vi "Creador ruta archivo para lectura continua.vi"(4 "error in (no error)":errorcluster, 7 "Datos de Nueva Adquisición In":T1={"Equipo a Utilizar"=enum."TDS 2012B Osciloscope", "Montura"=enum."Motor Bipolar", "Datos Zaber"={"Sentido de Adquisición"=FALSE, "Comenzar Desde Home?"=FALSE, "Distancia a recorrer (um)"=0.0, "Pasos motor"=0, "Distancia entre Lecturas (um)"=0.0, "Puerto"=""}, "Datos Bipolar/Unipolar"={"Puerto COM"="", "Pasos entre Lecturas"=0, "Numero de lecturas"=0, "Sentido del motor"=TRUE}, "Datos Archivo"={"Ruta Archivo"=path "", "Nombre de Prueba"=""}, "Datos actuales"={"Montura"="", "Equipo"="", "Posición Actual"="", "Distancia Total a recorrer"="", "distancia Entre lecturas"="", "Pasos entre lecturas"=""}, "Datos a Guardar In"={"Datos Cursor Tektronix"="", "Datos Lokin"="", "Posición Cero"=0.0, "Posición Actual"=0.0}, "Datos Osciloscopio"={"Sesión Visa Osciloscopio"="Tektronix_TDS2012C", "Tipo de Adquisición"=enum."Voltaje Pico Pico", "Canal a Utilizar"=enum."Canal 1", "Parametros de Adquisición"=enum."Una Muestra", "Número Promedio"=2}, "Datos Lock In"={"Visa Lock in"="Tektronix_TDS2012C"}} {"Datos Osciloscopio"."Número Promedio" min=2 max=20; "Datos a Guardar In"."Posición Actual" format="%#_10f"; "Datos a Guardar In"."Posición Cero" format="%#_10f"; "Datos Bipolar/Unipolar"."Numero de lecturas" max=910098 step=1}) -> (0 "error out":errorcluster, 3 "Datos de Nueva Adquisición out":T1={"Equipo a Utilizar"=enum."TDS 2012B Osciloscope", "Montura"=enum."Motor Bipolar", "Datos Zaber"={"Sentido de Adquisición"=FALSE, "Comenzar Desde Home?"=FALSE, "Distancia a recorrer (um)"=0.0, "Pasos motor"=0, "Distancia entre Lecturas (um)"=0.0, "Puerto"=""}, "Datos Bipolar/Unipolar"={"Puerto COM"="", "Pasos entre Lecturas"=0, "Numero de lecturas"=0, "Sentido del motor"=TRUE}, "Datos Archivo"={"Ruta Archivo"=path "", "Nombre de Prueba"=""}, "Datos actuales"={"Montura"="", "Equipo"="", "Posición Actual"="", "Distancia Total a recorrer"="", "distancia Entre lecturas"="", "Pasos entre lecturas"=""}, "Datos a Guardar In"={"Datos Cursor Tektronix"="", "Datos Lokin"="", "Posición Cero"=0.0, "Posición Actual"=0.0}, "Datos Osciloscopio"={"Sesión Visa Osciloscopio"="Tektronix_TDS2012C", "Tipo de Adquisición"=enum."Voltaje Pico Pico", "Canal a Utilizar"=enum."Canal 1", "Parametros de Adquisición"=enum."Una Muestra", "Número Promedio"=2}, "Datos Lock In"={"Visa Lock in"="Tektronix_TDS2012C"}} {"Datos Osciloscopio"."Número Promedio" min=2 max=20; "Datos a Guardar In"."Posición Actual" format="%#_10f"; "Datos a Guardar In"."Posición Cero" format="%#_10f"; "Datos Bipolar/Unipolar"."Numero de lecturas" max=910098 step=1})   [LabVIEW 2020]
doc: "Este Vi Crea una ruta para el proyecto RPS utilizando fecha hora y nombre de prueba"
uses:
  Type Definitions/Asistente de adquisicion Cluster.ctl
  Type Definitions/Datos a Guardar.ctl
  Type Definitions/datos osciloscopio.ctl
  Type Definitions/Datos Zaber.ctl
  Type Definitions/parametros motores.ctl
  H:/Mi unidad/Departamento de Ingenieria/Investigadores/Gabriel Ramos/Proyecto Monturas v13/LV Source/Type Definitions/Tipos de montura.ctl
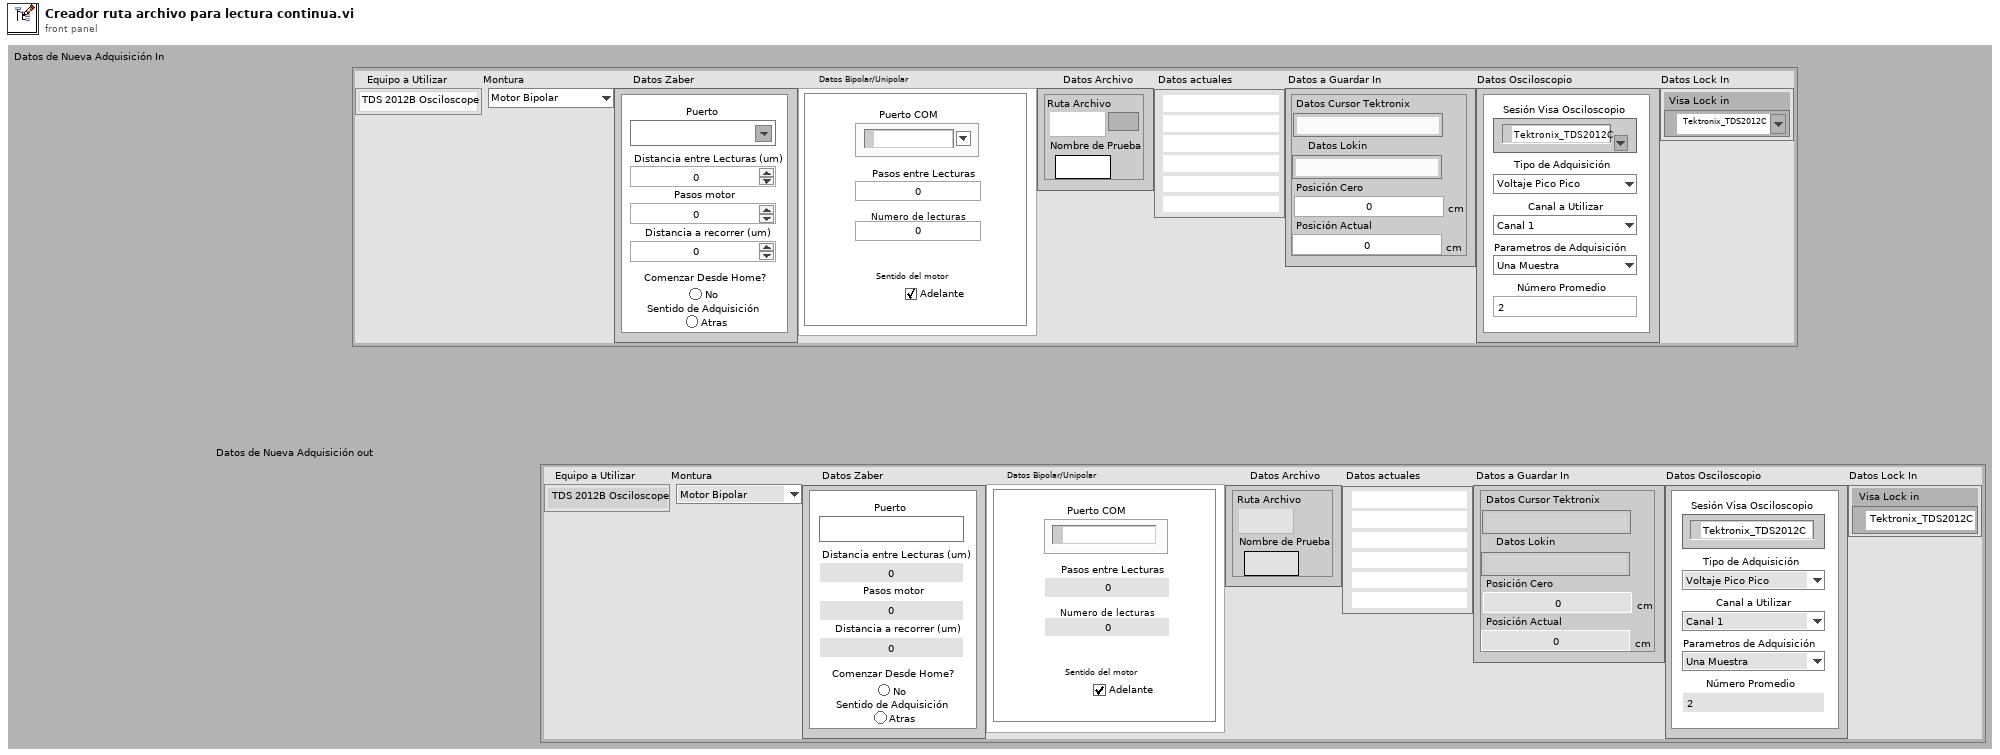
[diagram p1: front panel]
types:
  T1 = typedef "Asistente de adquisicion Cluster.ctl" = cluster{"Equipo a Utilizar":enum16{"SR830 Lock In", "TDS 2012B Osciloscope"}, "Montura":T2, "Datos Zaber":T3, "Datos Bipolar/Unipolar":T4, "Datos Archivo":cluster{"Ruta Archivo":path, "Nombre de Prueba":string}, "Datos actuales":cluster{"Montura":string, "Equipo":string, "Posición Actual":string, "Distancia Total a recorrer":string, "distancia Entre lecturas":string, "Pasos entre lecturas":string}, "Datos a Guardar In":T5, "Datos Osciloscopio":T6, "Datos Lock In":cluster{"Visa Lock in":refnum<visa-resource-name>}}
  T2 = typedef "Tipos de montura.ctl" = enum16{"Zaber T-LSR450B", "Zaber-T-LSR300B", "Zaber-T-LSRxxx", "Motor Bipolar", "Motor Unipolar"}
  T3 = typedef "Datos Zaber.ctl" = cluster{"Sentido de Adquisición":bool, "Comenzar Desde Home?":bool, "Distancia a recorrer (um)":dbl, "Pasos motor":i32, "Distancia entre Lecturas (um)":dbl, "Puerto":refnum<visa-resource-name>}
  T4 = typedef "parametros motores.ctl" = cluster{"Puerto COM":refnum<visa-resource-name>, "Pasos entre Lecturas":u16, "Numero de lecturas":u32, "Sentido del motor":bool}
  T5 = typedef "Datos a Guardar.ctl" = cluster{"Datos Cursor Tektronix":string, "Datos Lokin":string, "Posición Cero":dbl[unit], "Posición Actual":dbl[unit]}
  T6 = typedef "datos osciloscopio.ctl" = cluster{"Sesión Visa Osciloscopio":refnum<visa-resource-name>, "Tipo de Adquisición":enum16{"Voltaje Pico Pico", "Voltaje RMS", "Cursor Tiempo"}, "Canal a Utilizar":enum16{"Canal 1", "Canal 2", "Canal 1 y 2"}, "Parametros de Adquisición":enum16{"Una Muestra", "Promedio"}, "Número Promedio":i32}
  T7 = enum16{"open", "replace", "create", "open or create", "replace or create", "replace or create with confirmation"}
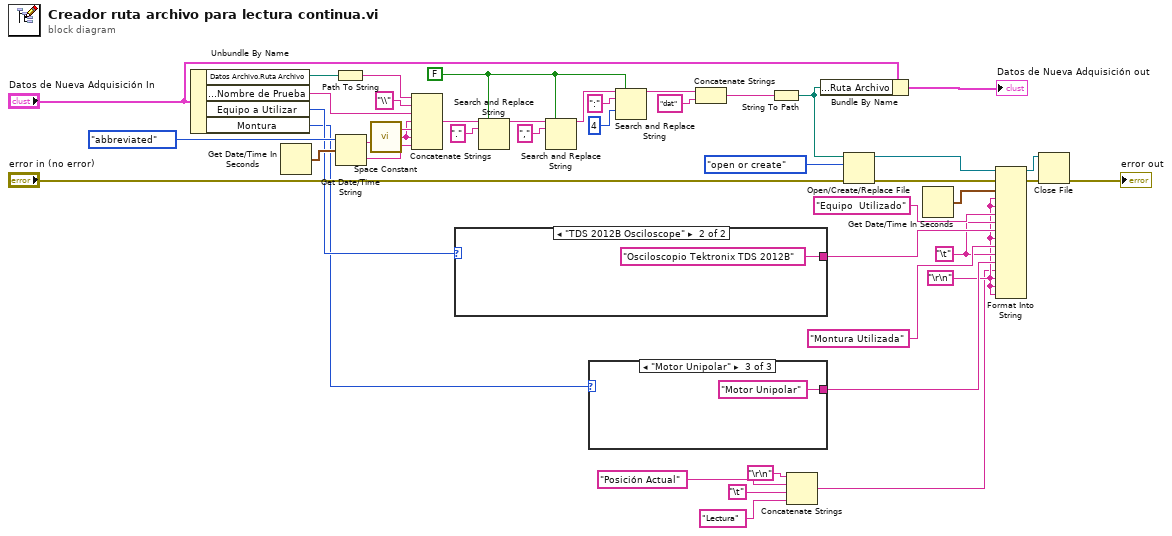
[diagram p0: block diagram]
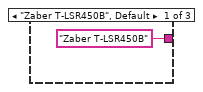
[diagram p2: hidden frame]
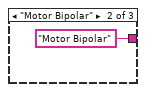
[diagram p3: hidden frame]
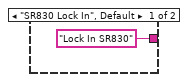
[diagram p4: hidden frame]
diagram:
  w6 = "\r\n"
  w15 = "\t"
  w43 = FALSE ("replace all? (F)")
  n1 = Unbundle By Name("Datos de Nueva Adquisición In") -> ("Datos Archivo.Ruta Archivo"=w21:path, "Datos Archivo.Nombre de Prueba"=w22:string, "Equipo a Utilizar"=w18:enum16{"SR830 Lock In", "TDS 2012B Osciloscope"}, "Montura"=w14:T2)
  n2 = Get Date/Time In Seconds() -> (seconds since 1Jan1904=w33:timestamp)
  n3 = Path To String(path=w21) -> (string=w31:string)
  n4 = Get Date/Time String(date format (0)=enum16{"short", "long", "abbreviated"}."abbreviated", seconds (now)=w33) -> (date string=w29:string, time string=w27:string)  [unwired: 1 in]
  n5 = call <vilib>:"Space Constant.vi"() -> ("String"=w28:string)
  n6 = Concatenate Strings(w31, "\\" ("string"), w22, w28, w29, w28, w27) -> (w35:string)
  n7 = case shown="\"TDS 2012B Osciloscope\"" w18 {
    tunnel: ["Lock In SR830" "Osciloscopio Tektronix TDS 2012B"] -> w17
    frame "SR830 Lock In", Default {
    }
    frame "TDS 2012B Osciloscope" {
    }
  }
  n8 = Search and Replace String(replace all?=w43, input string=w35, search string=".") -> (result string=w39:string)  [unwired: 5 in, 3 out]
  n9 = Search and Replace String(replace all?=w43, input string=w39, search string=",") -> (result string=w40:string)  [unwired: 5 in, 3 out]
  n10 = case shown="\"Motor Unipolar\"" w14 {
    tunnel: ["Zaber T-LSR450B" "Motor Bipolar" "Motor Unipolar"] -> w13
    frame "Zaber T-LSR450B", Default {
    }
    frame "Motor Bipolar" {
    }
    frame "Motor Unipolar" {
    }
  }
  n11 = Search and Replace String(replace all?=w43, input string=w40, search string=":", offset=4 ("offset (0)")) -> (result string=w42:string)  [unwired: 4 in, 3 out]
  n12 = Concatenate Strings(w42, "dat" ("string")) -> (w32:string)
  n13 = String To Path(string=w32) -> (path=w8:path)
  n14 = Concatenate Strings("\r\n", "Posición Actual" ("string"), "\t", "Lectura" ("string")) -> (w2:string)
  n15 = Bundle By Name(cluster="Datos de Nueva Adquisición In", "Datos Archivo.Ruta Archivo"=w8) -> (→"Datos de Nueva Adquisición out":T1)
  n16 = Open/Create/Replace File(file path (use dialog)=w8, error in="error in (no error)", operation (0:open)=T7."open or create") -> (refnum out=w24:refnum<file>, error out=w25:errorcluster)  [unwired: 3 in, 1 out]
  n17 = Get Date/Time In Seconds() -> (seconds since 1Jan1904=w20:timestamp)
  n18 = Format Into String(initial string=w24, error in=w25, w20, w6, w6, "Equipo  Utilizado" ("input 4"), w15, w17, w6, "Montura Utilizada" ("input 8"), w15, w13, w2, w6, w6, w6) -> (resulting string=w12:refnum<file>, error out=w10:errorcluster)  [unwired: 1 in]
  n19 = Close File(refnum=w12, error in=w10) -> (error out=→"error out":errorcluster)  [unwired: 1 out]
